vi "MH_LoadHistGraph.vi"(8 "ErrIn(No Err)":errorcluster caption="entrée d'erreur (pas d'erreur)", 11 "Rate Mode":bool) -> (0 "ErrOut":errorcluster caption="sortie d'erreur", 1 "Graph":refnum<vi>, 2 "Dat":refnum<vi>, 3 "ViRef":refnum<vi>, 4 "MaxT ref":refnum<vi>, 5 "Avg ref":refnum<vi>)   [LabVIEW 2019]
panel:
  out "Exécution:État":T1(ring)
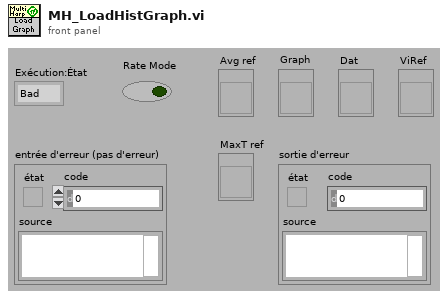
[diagram p1: front panel]
types:
  T1 = enum32{"Bad", "Idle", "Run top level", "Running"}
  T2 = enum32{"Invalid", "Standard", "Closed", "Hidden", "Minimized", "Maximized"}
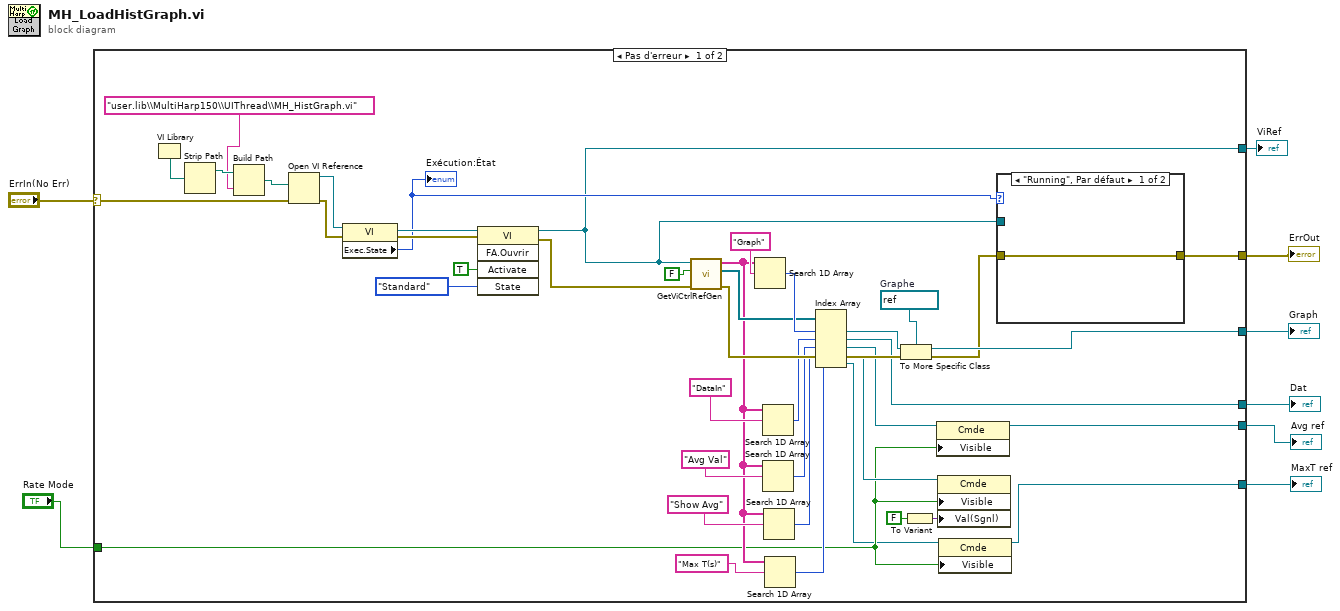
[diagram p0: block diagram]
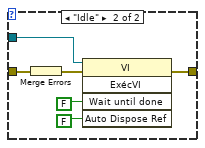
[diagram p2: hidden frame]
diagram:
  n1 = case shown="Pas d'erreur" "ErrIn(No Err)" {
    selector: "ErrIn(No Err)" -> [w37 w58]
    tunnel: [w43 w58] -> w7
    tunnel: [w46 _] -> w6
    tunnel: [w25 _] -> w5
    tunnel: [w24 _] -> w4
    tunnel: "Rate Mode" -> [w11 _]
    tunnel: [w16 _] -> w2
    tunnel: [w9 _] -> w1
    frame No Error {
      w45 = refnum<vi> refnum  # Graphe
      n2 = VI Library() -> (path=w38:path)
      n3 = Strip Path(path=w38) -> (stripped path=w31:path)  [unwired: 1 out]
      n4 = Build Path(base path=w31, name or relative path="user.lib\\MultiHarp150\\UIThread\\MH_HistGraph.vi" ("NomFichier")) -> (appended path=w30:path)
      n5 = Open VI Reference(vi path=w30, error in (no error)=w37) -> (vi reference=w35:refnum<vi>, error out=w34:errorcluster)  [unwired: 4 in]
      n6 = property class="VI"(reference=w35, error in=w34) -> (reference out=w32:refnum<vi>, error out=w33:errorcluster, "Exec.State"=w28:T1)
      "Exécution:État" <- w28
      n7 = invoke class="VI" method="FA.Ouvrir"(reference=w32, error in=w33, "Activate"=TRUE ("Activer ?"), "State"=T2."Standard" ("État")) -> (reference out=w24:refnum<vi>, error out=w36:errorcluster)  [unwired: 1 in, 3 out]
      n8 = call <userlib>:"GetViCtrlRefGen.vi"("ErrorIn(No Error)"=w36, "InclTabCTrl"=FALSE, "VIRef"=w24) -> ("sortie d'erreur"=w41:errorcluster, "ControlsRefs"=w42:refnum<vi>[], "ControlsNames"=w13:string[])  [unwired: 6 in]
      n9 = Search 1D Array(1D array=w13, element="Graph" ("élément")) -> (index of element=w48:i32)  [unwired: 1 in]
      n10 = Search 1D Array(1D array=w13, element="DataIn" ("élément")) -> (index of element=w26:i32)  [unwired: 1 in]
      n11 = Search 1D Array(1D array=w13, element="Avg Val" ("élément")) -> (index of element=w19:i32)  [unwired: 1 in]
      n12 = Search 1D Array(1D array=w13, element="Show Avg" ("élément")) -> (index of element=w15:i32)  [unwired: 1 in]
      n13 = Search 1D Array(1D array=w13, element="Max T(s)" ("élément")) -> (index of element=w12:i32)  [unwired: 1 in]
      n14 = Index Array(array=w42, index #1=w48, index #2=w26, index #3=w19, index #4=w15, index #5=w12) -> (element #1=w47:refnum<vi>, element #2=w25:refnum<vi>, element #3=w21:refnum<vi>, element #4=w20:refnum<vi>, element #5=w10:refnum<vi>)
      n15 = To More Specific Class(target class=w45, reference=w47, error in=w41) -> (specific class reference=w46:refnum<vi>, error out=w44:errorcluster)
      n16 = To Variant(anything=FALSE) -> (Variant=w18:variant)
      n17 = property class="Cmde"(reference=w21, "Visible"=w11) -> (reference out=w16:refnum<vi>)  [unwired: 1 in, 1 out]
      n18 = property class="Cmde"(reference=w20, "Visible"=w11, "Val(Sgnl)"=w18) -> ()  [unwired: 1 in, 2 out]
      n19 = property class="Cmde"(reference=w10, "Visible"=w11) -> (reference out=w9:refnum<vi>)  [unwired: 1 in, 1 out]
      n20 = case shown="\"Running\", Par défaut" w28 {
        tunnel: w44 -> [w51 w55]
        tunnel: [w51 w53] -> w43
        tunnel: w24 -> [_ w52]
        frame "Running", Default {
        }
        frame "Idle" {
          n21 = Merge Errors(w55) -> (w54:errorcluster)
          n22 = invoke class="VI" method="ExécVI"(reference=w52, error in=w54, "Wait until done"=FALSE ("Attendre la fin"), "Auto Dispose Ref"=FALSE ("Supprimer la référence automatiquement")) -> (error out=w53:errorcluster)  [unwired: 1 in, 4 out]
        }
      }
    }
    frame Error {
    }
  }
  "ErrOut" <- w7
  "Graph" <- w6
  "Dat" <- w5
  "ViRef" <- w4
  "Avg ref" <- w2
  "MaxT ref" <- w1
